vi "Throw Error.vi"(8 "error in":errorcluster, 9 "VeriStand Error In":T1, 10 "Key":string, 11 "Item Ref in":T2 format="%.0x") -> (0 "error out":errorcluster, 3 "Item Ref out":T2=18446744073709551615 format="%.0x")   [LabVIEW 2020, in "VeriStand Error API.lvlib"]
doc: "<B>Throw Error</B> adds an error the VeriStand error handler with the key specified."
uses:
  VeriStand Error API.lvlib
  C:/NetCoreDLL/NationalInstruments.VeriStand.SystemStorage.dll
  NetCoreDLL/NationalInstruments.VeriStand.SystemStorage.dll
  <vilib>/NI VeriStand/Custom Device API/Custom Device API.lvlib
  <vilib>/NI VeriStand/Custom Device API/Custom Device Item Ref.ctl
  VeriStand Error.ctl
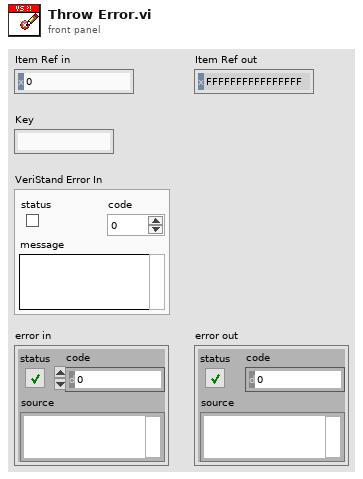
[diagram p1: front panel]
types:
  T1 = typedef "VeriStand Error API.lvlib/VeriStand Error.ctl" = cluster{"status":bool, "code":i32, "message":string}
  T2 = typedef "Custom Device API.lvlib/Custom Device Item Ref.ctl" = u64
  T3 = typedef "Custom Device API.lvlib/Custom Device Pointer.ctl" = refnum<k39>
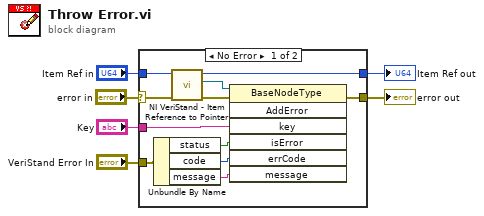
[diagram p0: block diagram]
diagram:
  n1 = case shown="No Error" "error in" {
    selector: "error in" -> [w17 w19]
    tunnel: "Item Ref in" -> [w16 w18]
    tunnel: [w15 w18] -> w4
    tunnel: [w12 w19] -> w3
    tunnel: "Key" -> [w11 _]
    tunnel: "VeriStand Error In" -> [w7 _]
    frame No Error {
      n2 = Unbundle By Name(w7) -> ("status"=w10:bool, "code"=w9:i32, "message"=w8:string)
      n3 = call <vilib>:"NI VeriStand - Item Reference to Pointer.vi"("error in (no error)"=w17, "Item Ref in"=w16) -> ("error out"=w13:errorcluster, "Node Pointer"=w14:T3, "Item Ref out"=w15:T2)  [unwired: 6 in, 1 out]
      n4 = invoke class="BaseNodeType" method="AddError"(reference=w14, error in=w13, "key"=w11, "isError"=w10, "errCode"=w9, "message"=w8) -> (error out=w12:errorcluster)  [unwired: 1 in, 6 out]
    }
    frame Error {
    }
  }
  "Item Ref out" <- w4
  "error out" <- w3
